vi "FGV_ADQ.vi"(8 "error in (no error)":errorcluster, 9 "Com_Escribir_IN":T1, 10 "SM_IN":T2=enum."Stop", 11 "SET/GET":enum16{"SET", "GET"}(ring)) -> (0 "error out":errorcluster, 1 "Com_Escribir_OUT":T1, 2 "SM_OUT":T2=enum."Stop")   [LabVIEW 2026]
uses:
  Ctrl_Estados.ctl
  Control/Ctrl_EscrituraComandos.ctl
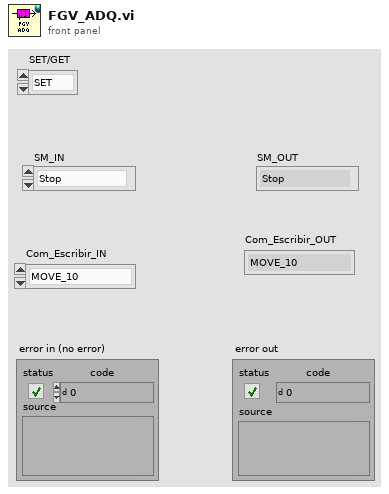
[diagram p1: front panel]
types:
  T1 = typedef "Ctrl_EscrituraComandos.ctl" = enum16{"MOVE_10", "HOME_TO"}
  T2 = typedef "Ctrl_Estados.ctl" = enum16{"LogData", "Idle", "Stop", "Show_Dashboard", "Reconnect", "Log_Data_All", "Start", "WRITE_DATA", "SEND_COM"}
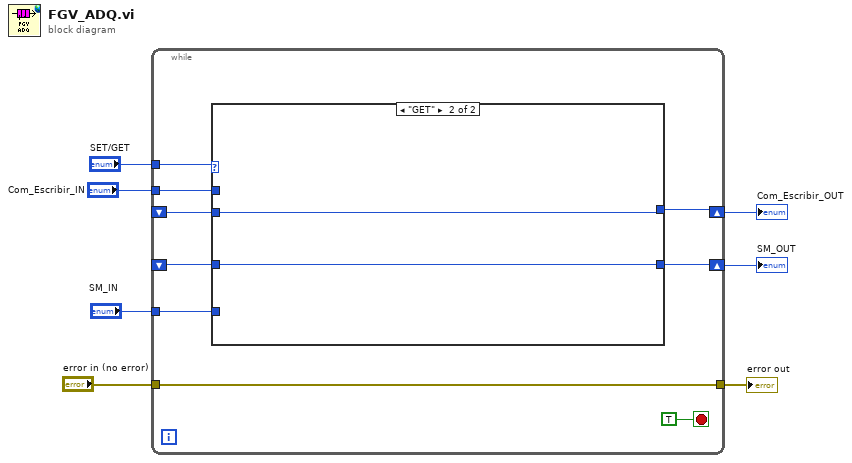
[diagram p0: block diagram]
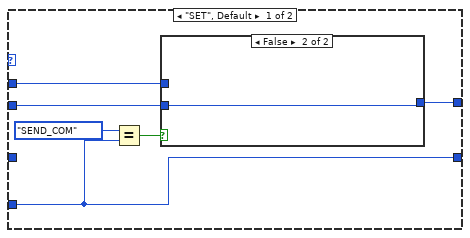
[diagram p2: hidden frame]
diagram:
  n1 = while {
    tunnel: "SM_IN" -> [w12]
    tunnel: "SET/GET" -> [w15]
    shift-right: [w13] -> w5
    shift-left: _ -> [w14]
    tunnel: "error in (no error)" -> [w11]
    tunnel: [w11] -> w3
    shift-right: [w10] -> w1
    shift-left: _ -> [w8]
    tunnel: "Com_Escribir_IN" -> [w9]
    stop <- TRUE stop-if-true
    n2 = case shown="\"GET\"" w15 {
      tunnel: [w22 w25] -> w13
      tunnel: w14 -> [_ w25]
      tunnel: w12 -> [w22 _]
      tunnel: [w18 w26] -> w10
      tunnel: w9 -> [w19 _]
      tunnel: w8 -> [w17 w26]
      frame "SET", Default {
        n3 = Equal?(x=Ctrl_Estados."SEND_COM", y=w22) -> (x = y?=w21:bool)
        n4 = case shown="False" w21 {
          tunnel: w19 -> [w23 _]
          tunnel: [w23 w24] -> w18
          tunnel: w17 -> [_ w24]
          frame True {
          }
          frame False {
          }
        }
      }
      frame "GET" {
      }
    }
  }
  "SM_OUT" <- w5
  "error out" <- w3
  "Com_Escribir_OUT" <- w1
